vi "Spatial Dual Decode Packet 58 (SubVI).vi"(8 "SGL Precision":i16=6, 10 "Packet 58 Bytes In":u8[](array[numeric])) -> (0 "Channel Data Type":string[](array[string])=["Float", "Float", "Float"], 1 "Channel Units":string[](array[string])=["m/s/s", "m/s/s", "m/s/s"], 2 "Data":string[](array[string]), 3 "Channel Names":string[](array[string])=["Acc X", "Acc Y", "Acc Z"], 4 "Packet 58 Decoded Data Cluster":T1)   [LabVIEW 2019, in "SpatialDual_Parsers.lvlib"]
uses:
  SpatialDual_Parsers.lvlib
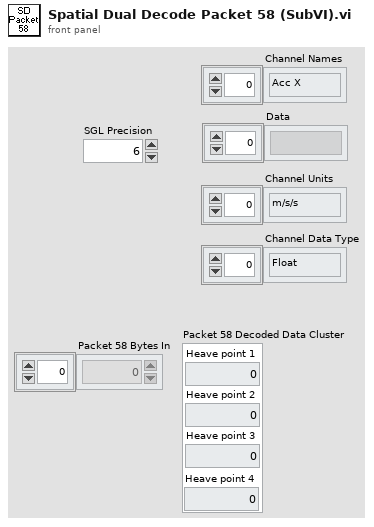
[diagram p1: front panel]
types:
  T1 = cluster{"Heave point 1":sgl, "Heave point 2":sgl, "Heave point 3":sgl, "Heave point 4":sgl}
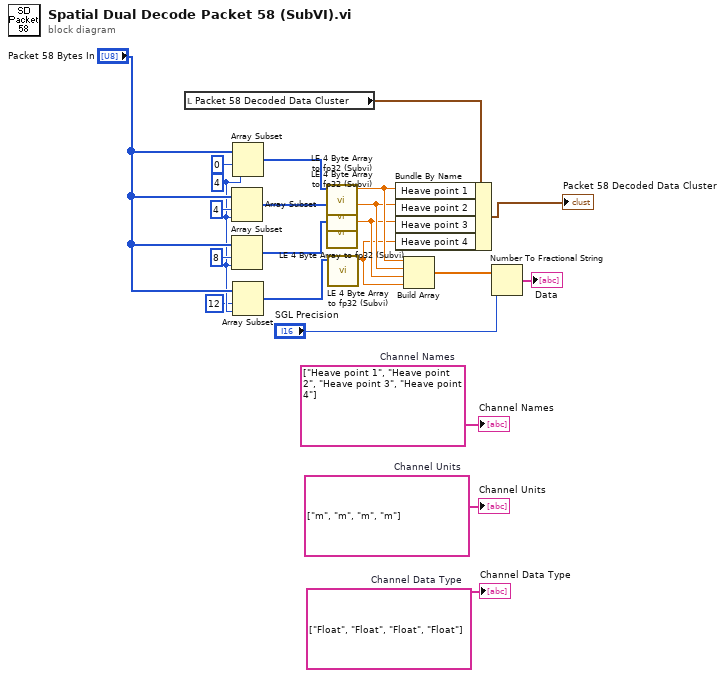
[diagram p0: block diagram]
diagram:
  w6 = string[] ["Float", "Float", "Float", "Float"]  # Channel Data Type
  w7 = string[] ["m", "m", "m", "m"]  # Channel Units
  w8 = string[] ["Heave point 1", "Heave point 2", "Heave point 3", "Heave point 4"]  # Channel Names
  w4 = 4 ("length")
  n1 = local read "Packet 58 Decoded Data Cluster"() -> (w22:T1)
  n2 = Array Subset(array="Packet 58 Bytes In", index=4, length=w4) -> (w16:u8[])
  n3 = Array Subset(array="Packet 58 Bytes In", index=8, length=w4) -> (w17:u8[])
  n4 = Array Subset(array="Packet 58 Bytes In", index=0, length=w4) -> (w15:u8[])
  n5 = Array Subset(array="Packet 58 Bytes In", index=12, length=w4) -> (w2:u8[])
  n6 = call "LE 4 Byte Array to fp32 (Subvi).vi"("4 Bytes in"=w15) -> ("fp32 Out"=w14:sgl)  [unwired: 8 in]
  n7 = call "LE 4 Byte Array to fp32 (Subvi).vi"("4 Bytes in"=w16) -> ("fp32 Out"=w13:sgl)  [unwired: 8 in]
  n8 = call "LE 4 Byte Array to fp32 (Subvi).vi"("4 Bytes in"=w17) -> ("fp32 Out"=w12:sgl)  [unwired: 8 in]
  n9 = call "LE 4 Byte Array to fp32 (Subvi).vi"("4 Bytes in"=w2) -> ("fp32 Out"=w1:sgl)  [unwired: 8 in]
  n10 = Bundle By Name(cluster=w22, "Heave point 1"=w14, "Heave point 2"=w13, "Heave point 3"=w12, "Heave point 4"=w1) -> (→"Packet 58 Decoded Data Cluster":T1)
  n11 = Build Array(w14, w13, w12, w1) -> (w11:sgl[])
  n12 = Number To Fractional String(number=w11, precision (6)="SGL Precision") -> (F-format string=→"Data":string[])  [unwired: 2 in]
  "Channel Names" <- w8
  "Channel Units" <- w7
  "Channel Data Type" <- w6
